vi "AlliGator Use Phasor Plot Segment Extremities as References.vi"(8 "Error In":errorcluster, 9 "Phasor Frequency":dbl[unit], 11 "Image Points":T2[](array[typedef])) -> (0 "error out":errorcluster, 1 "Phasor 2":T1, 2 "Phasor 1":T1)   [LabVIEW 2021, in "AlliGator Phasor Plot.lvlib"]
doc: "Defines the references as the extremities of the user-drawn segment in the Phasor Plot image."
uses:
  AlliGator Phasor Plot.lvlib
  Image/Image Point.ctl
  Phasor/Phasor (g, s).ctl
  Phasor Ratio/AlliGator Phasor Ratio.lvlib
  Image/Image.lvlib
  Phasor/Phasor.lvlib
panel:
  # "see the AlliGator License on the block diagram (Ctrl+E or Window:Show Block Diagram)"
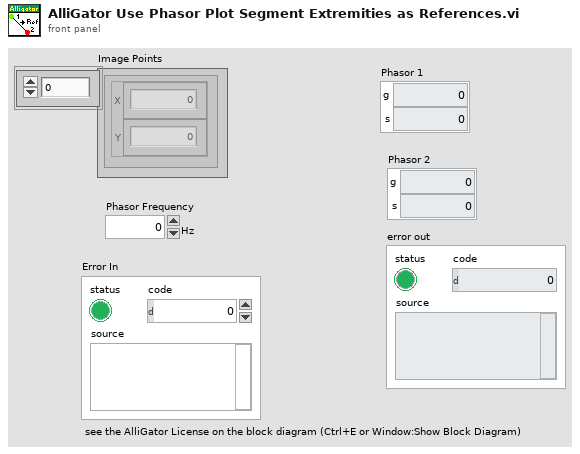
[diagram p1: front panel]
types:
  T1 = typedef "Phasor.lvlib/Phasor (g, s).ctl" = cluster{"g":dbl, "s":dbl}
  T2 = typedef "Image.lvlib/Image Point.ctl" = cluster{"X":i32, "Y":i32}
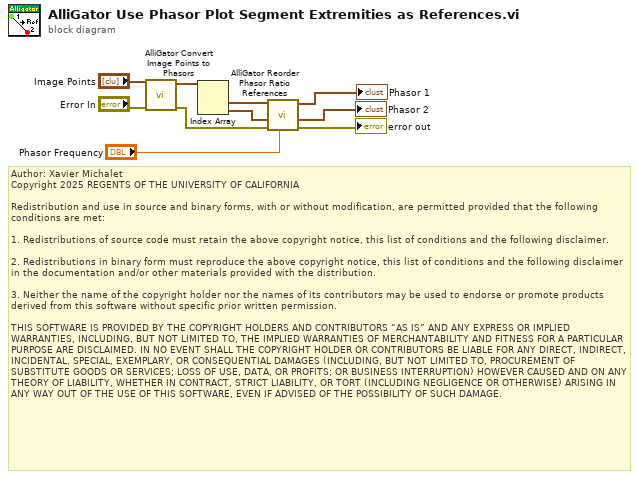
[diagram p0: block diagram]
diagram:
  # "Author: Xavier Michalet\nCopyright 2025 REGENTS OF THE UNIVERSITY OF CALIFORNIA\n\nRedistribution and use in source and binary forms, with or without modification, are permitted provided that the following conditions are met:\n\n1. Redistributions of source code must retain the above copyright notice, this list of conditions and the following disclaimer.\n\n2. Redistributions in binary form must reproduce the above copyright notice, this list of conditions and the following disclaimer in the documentation and/or other materials provided with the distribution.\n\n3. Neither the name of the copyright holder nor the names of its contributors may be used to endorse or promote products derived from this software without specific prior written permission.\n\nTHIS SOFTWARE IS PROVIDED BY THE COPYRIGHT HOLDERS AND CONTRIBUTORS “AS IS” AND ANY EXPRESS OR IMPLIED WARRANTIES, INCLUDING, BUT NOT LIMITED TO, THE IMPLIED WARRANTIES OF MERCHANTABILITY AND FITNESS FOR A PARTICULAR PURPOSE ARE DISCLAIMED. IN NO EVENT SHALL THE COPYRIGHT HOLDER OR CONTRIBUTORS BE LIABLE FOR ANY DIRECT, INDIRECT, INCIDENTAL, SPECIAL, EXEMPLARY, OR CONSEQUENTIAL DAMAGES (INCLUDING, BUT NOT LIMITED TO, PROCUREMENT OF SUBSTITUTE GOODS OR SERVICES; LOSS OF USE, DATA, OR PROFITS; OR BUSINESS INTERRUPTION) HOWEVER CAUSED AND ON ANY THEORY OF LIABILITY, WHETHER IN CONTRACT, STRICT LIABILITY, OR TORT (INCLUDING NEGLIGENCE OR OTHERWISE) ARISING IN ANY WAY OUT OF THE USE OF THIS SOFTWARE, EVEN IF ADVISED OF THE POSSIBILITY OF SUCH DAMAGE."
  n1 = call "AlliGator Convert Image Points to Phasors.vi"("Error In"="Error In", "Image Points"="Image Points") -> ("Error Out"=w5:errorcluster, "Phasors"=w10:T1[])  [unwired: 8 in]
  n2 = Index Array(array=w10) -> (element #1=w7:T1, element #2=w6:T1)  [unwired: 2 in]
  n3 = call "AlliGator Reorder Phasor Ratio References.vi"("Phasor Frequency"="Phasor Frequency", "error in (no error)"=w5, "Phasor 2"=w6, "Phasor 1"=w7) -> ("error out"=→"error out":errorcluster, "Reference 2"=→"Phasor 2":T1, "Reference 1"=→"Phasor 1":T1)  [unwired: 3 in, 2 out]
